vi "Tree Manager.vi"(7 "Mode":T4, 9 "Alias":string, 10 "Init Settings In":T1={"Step Values"=[], "Only Execute When Test Running"=TRUE, "Reset Sequence When Test Starts"=TRUE, "Current Sequence ID"=0, "Total Iterations"=0, "Current Step Start Timestamp"=0.0, "Number of Sequence Steps"=0, "Num of Analog Channels"=0, "Num of Digital Channels"=0, "Delay Before Starting Sequence"=0.0, "Show UI"=FALSE, "Time Remaining"=0.0, "Test Running"=FALSE, "Pause Timestamp"=0.0, "Default Analog Values"=[], "Default Digital Values"=[]}, 11 "Init Refs":T3) -> (3 "Settings Out":T1={"Step Values"=[], "Only Execute When Test Running"=TRUE, "Reset Sequence When Test Starts"=TRUE, "Current Sequence ID"=0, "Total Iterations"=0, "Current Step Start Timestamp"=0.0, "Number of Sequence Steps"=0, "Num of Analog Channels"=0, "Num of Digital Channels"=0, "Delay Before Starting Sequence"=0.0, "Show UI"=FALSE, "Time Remaining"=0.0, "Test Running"=FALSE, "Pause Timestamp"=0.0, "Default Analog Values"=[], "Default Digital Values"=[]})   [LabVIEW 2020, in "Sequencer with Output Values.lvlib" / "Sequencer with Output Values.lvclass"]
uses:
  Sequencer with Output Values.lvclass
  Tree Manager Mode.ctl
  Control Refs.ctl
  Params.ctl
  Step Settings.ctl
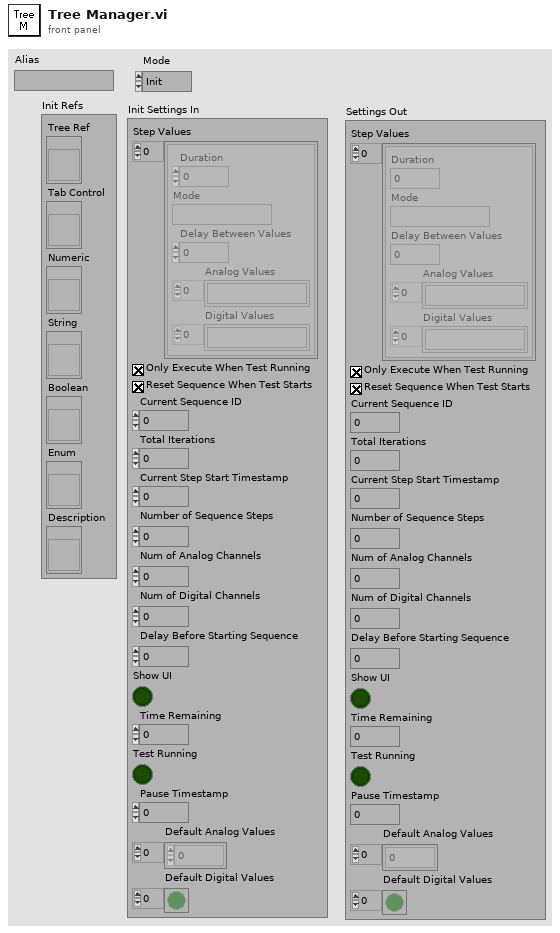
[diagram p1: front panel]
types:
  T1 = typedef "Sequencer with Output Values.lvlib/Sequencer with Output Values.lvclass/Params.ctl" = cluster{"Step Values":T2[], "Only Execute When Test Running":bool, "Reset Sequence When Test Starts":bool, "Current Sequence ID":u32, "Total Iterations":u32, "Current Step Start Timestamp":dbl, "Number of Sequence Steps":i32, "Num of Analog Channels":i32, "Num of Digital Channels":i32, "Delay Before Starting Sequence":dbl, "Show UI":bool, "Time Remaining":dbl, "Test Running":bool, "Pause Timestamp":dbl, "Default Analog Values":dbl[], "Default Digital Values":bool[]}
  T2 = typedef "Sequencer with Output Values.lvlib/Sequencer with Output Values.lvclass/Step Settings.ctl" = cluster{"Duration":dbl, "Mode":string, "Delay Between Values":dbl, "Analog Values":string[], "Digital Values":string[]}
  T3 = typedef "Sequencer with Output Values.lvlib/Sequencer with Output Values.lvclass/Control Refs.ctl" = cluster{"Tree Ref":refnum<vi>, "Tab Control":refnum<vi>, "Numeric":refnum<vi>, "String":refnum<vi>, "Boolean":refnum<vi>, "Enum":refnum<vi>, "Description":refnum<vi>}
  T4 = typedef "Sequencer with Output Values.lvlib/Sequencer with Output Values.lvclass/Tree Manager Mode.ctl" = enum16{"Init", "Tree Change", "Value Change", "Close"}
  T5 = typedef "Sequencer with Output Values.lvlib/Sequencer with Output Values.lvclass/Tree Item Settings.ctl" = cluster{"Indent Level":i32, "Data Type":T6, "Numeric Range":cluster{"Min":dbl, "Max":dbl, "Inc":dbl}, "Enum Values":string[], "Default Value":string}
  T6 = typedef "Sequencer with Output Values.lvlib/Sequencer with Output Values.lvclass/Data Type.ctl" = i16
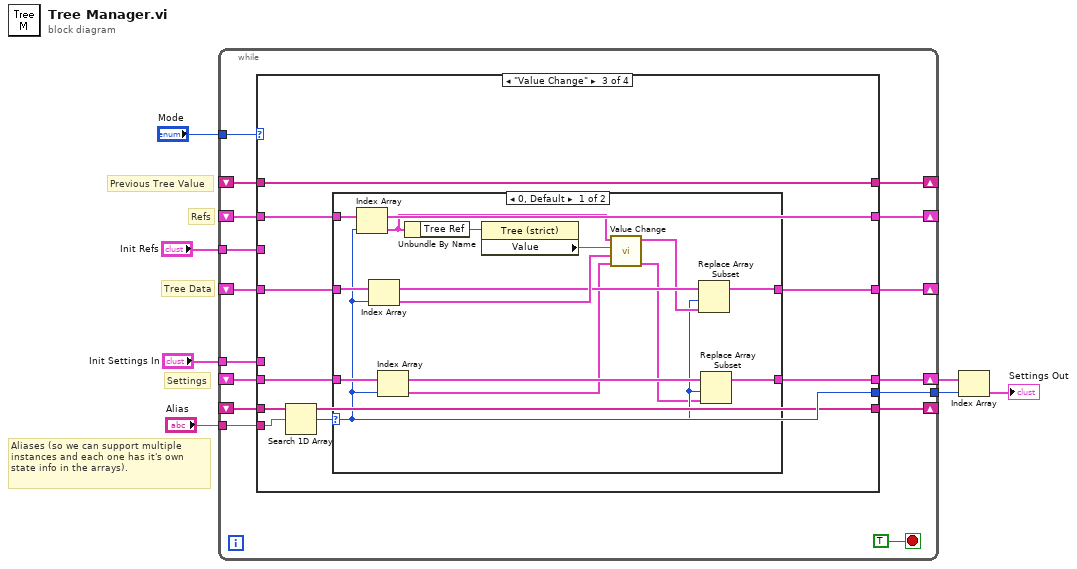
[diagram p0: block diagram]
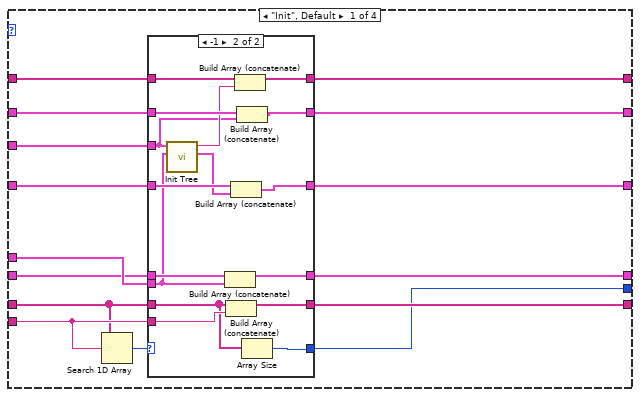
[diagram p2: hidden frame]
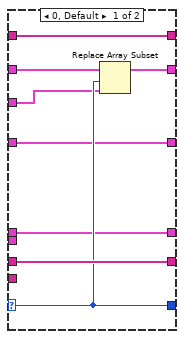
[diagram p3: hidden frame]
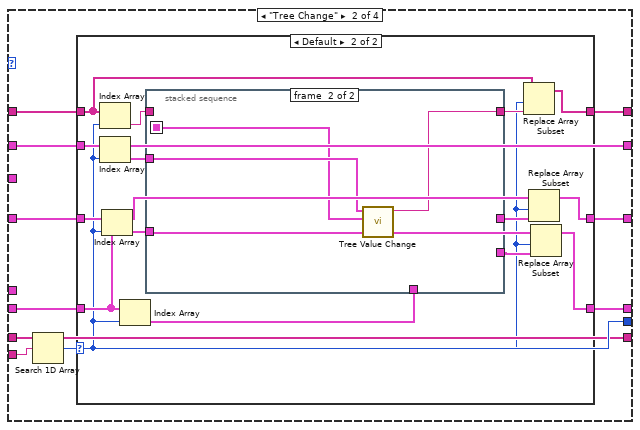
[diagram p4: hidden frame]
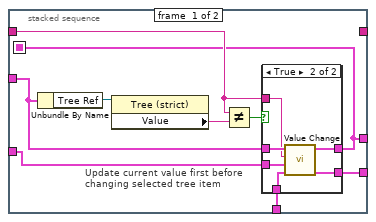
[diagram p6: hidden frame]
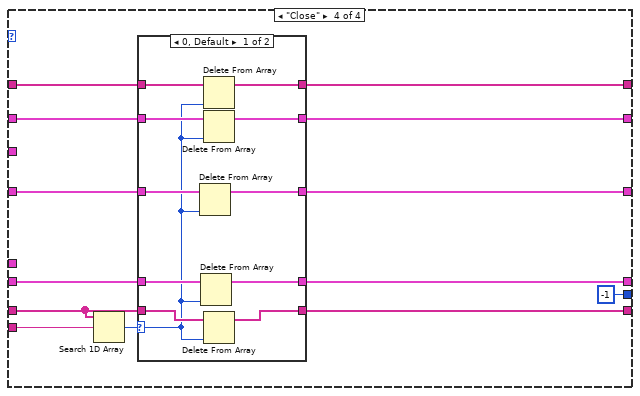
[diagram p9: hidden frame]
diagram:
  # "Aliases (so we can support multiple instances and each one has it's own state info in the arrays)."
  # "Previous Tree Value"
  # "Tree Data"
  # "Settings"
  # "Refs"
  n1 = while {
    tunnel: "Mode" -> [w23]
    tunnel: "Init Refs" -> [w22]
    tunnel: "Init Settings In" -> [w20]
    shift-right: [w19] -> _
    shift-left: _ -> [w18]
    shift-right: [w17] -> w4
    shift-left: _ -> [w16]
    shift-right: [w15] -> _
    shift-left: _ -> [w14]
    shift-right: [w13] -> _
    shift-left: _ -> [w12]
    tunnel: "Alias" -> [w11]
    shift-right: [w10] -> _
    shift-left: _ -> [w9]
    tunnel: [w8] -> w3
    stop <- TRUE stop-if-true
    n2 = case shown="\"Value Change\"" w23 {
      tunnel: w22 -> [w24 _ _ _]
      tunnel: w20 -> [w34 _ _ _]
      tunnel: [w26 w71 w118 w142] -> w19
      tunnel: w18 -> [w25 w71 w118 w143]
      tunnel: [w33 w67 w114 w138] -> w17
      tunnel: w16 -> [w32 w68 w116 w139]
      tunnel: [w30 w66 w115 w140] -> w15
      tunnel: w14 -> [w29 w72 w117 w141]
      tunnel: [w28 w70 w119 w144] -> w13
      tunnel: w12 -> [w27 w69 w119 w145]
      tunnel: w11 -> [w37 w65 w113 w147]
      tunnel: [w38 w63 w111 w136] -> w10
      tunnel: w9 -> [w35 w63 w111 w137]
      tunnel: [w31 w64 w112 -1 ("index of element")] -> w8
      frame "Init", Default {
        n3 = Search 1D Array(1D array=w35, element=w37) -> (index of element=w36:i32)  [unwired: 1 in]
        n4 = case shown="-1" w36 {
          selector: w36 -> [w43 _]
          tunnel: [w46 w62] -> w38
          tunnel: w37 -> [_ w61]
          tunnel: w35 -> [w46 w58]
          tunnel: w34 -> [_ w50]
          tunnel: [w39 w60] -> w33
          tunnel: w32 -> [w39 w59]
          tunnel: [w43 w57] -> w31
          tunnel: [w40 w56] -> w30
          tunnel: w29 -> [w40 w55]
          tunnel: [w42 w54] -> w28
          tunnel: w27 -> [w42 w53]
          tunnel: [w44 w52] -> w26
          tunnel: w25 -> [w45 w51]
          tunnel: w24 -> [w41 w47]
          frame 0, Default {
            n5 = Replace Array Subset(array=w45, new element=w41, index=w43) -> (w44:T3[])
          }
          frame -1 {
            n6 = call "Init Tree.vi"("Settings In"=w50, "Init Refs"=w47) -> ("Tree Data"=w48:cluster{string[], T5[]}, "Selected Tag"=w49:string)  [unwired: 8 in]
            n7 = Build Array (concatenate)(w59, w50) -> (w60:T1[])
            n8 = Build Array (concatenate)(w58, w61) -> (w62:string[])
            n9 = Build Array (concatenate)(w55, w48) -> (w56:cluster{string[], T5[]}[])
            n10 = Build Array (concatenate)(w53, w49) -> (w54:string[])
            n11 = Build Array (concatenate)(w51, w47) -> (w52:T3[])
            n12 = Array Size(array=w58) -> (size(s)=w57:i32)
          }
        }
      }
      frame "Tree Change" {
        n13 = Search 1D Array(1D array=w63, element=w65) -> (index of element=w64:i32)  [unwired: 1 in]
        n14 = case shown="Default" w64 {
          selector: w64 -> [_ w77]
          tunnel: w72 -> [w74 w82]
          tunnel: w71 -> [_ w90]
          tunnel: [w75 w83] -> w70
          tunnel: w69 -> [w75 w85]
          tunnel: w68 -> [w73 w79]
          tunnel: [w73 w76] -> w67
          tunnel: [w74 w80] -> w66
          frame -1 {
          }
          frame Default {
            n15 = Index Array(array=w85, index=w77) -> (element=w88:string)
            n16 = Index Array(array=w90, index=w77) -> (element=w89:T3)
            n17 = Index Array(array=w82, index=w77) -> (element=w87:cluster{string[], T5[]})
            n18 = Index Array(array=w79, index=w77) -> (element=w86:T1)
            n19 = stacked-sequence {
              seq-local: [w91 _] -> [_ w108]
              tunnel: w87 -> [w94 _]
              tunnel: w89 -> [w98 w110]
              tunnel: [_ w109] -> w84
              tunnel: w88 -> [w95 _]
              tunnel: w86 -> [w93 _]
              tunnel: [w92 _] -> w78
              tunnel: [w91 _] -> w81
              frame #0 {
                # "Update current value first before changing selected tree item"
                n20 = Unbundle By Name(w98) -> ("Tree Ref"=w99:refnum<vi>)
                n21 = property class="Tree (strict)"(reference=w99) -> ("Value"=w97:string)  [unwired: 1 in, 2 out]
                n22 = Not Equal?(x=w95, y=w97) -> (x != y?=w96:bool)
                n23 = case shown="True" w96 {
                  tunnel: w98 -> [_ w107]
                  tunnel: w95 -> [_ w106]
                  tunnel: w94 -> [w101 w105]
                  tunnel: w93 -> [w100 w104]
                  tunnel: [w101 w103] -> w91
                  tunnel: [w100 w102] -> w92
                  frame False {
                  }
                  frame True {
                    n24 = call "Value Change.vi"("Settings In"=w104, "Tree Data"=w105, "Tree Tag"=w106, "Init Refs"=w107) -> ("Settings Out"=w102:T1, "Tree Data out"=w103:cluster{"Tag":string[], "Settings":T5[]})  [unwired: 6 in]
                  }
                }
              }
              frame #1 {
                n25 = call "Tree Value Change.vi"("Tree Data"=w108, "Init Refs"=w110) -> ("Value"=w109:string)  [unwired: 9 in]
              }
            }
            n26 = Replace Array Subset(array=w85, new element=w84, index=w77) -> (w83:string[])
            n27 = Replace Array Subset(array=w82, new element=w81, index=w77) -> (w80:cluster{string[], T5[]}[])
            n28 = Replace Array Subset(array=w79, new element=w78, index=w77) -> (w76:T1[])
          }
        }
      }
      frame "Value Change" {
        n29 = Search 1D Array(1D array=w111, element=w113) -> (index of element=w112:i32)  [unwired: 1 in]
        n30 = case shown="0, Default" w112 {
          selector: w112 -> [w122 _]
          tunnel: w118 -> [w130 _]
          tunnel: w117 -> [w128 w134]
          tunnel: w116 -> [w125 w133]
          tunnel: [w126 w134] -> w115
          tunnel: [w124 w133] -> w114
          frame 0, Default {
            n31 = Index Array(array=w130, index=w122) -> (element=w123:T3)
            n32 = Index Array(array=w128, index=w122) -> (element=w129:cluster{string[], T5[]})
            n33 = Index Array(array=w125, index=w122) -> (element=w121:T1)
            n34 = Unbundle By Name(w123) -> ("Tree Ref"=w132:refnum<vi>)
            n35 = property class="Tree (strict)"(reference=w132) -> ("Value"=w131:string)  [unwired: 1 in, 2 out]
            n36 = call "Value Change.vi"("Settings In"=w121, "Tree Data"=w129, "Tree Tag"=w131, "Init Refs"=w123) -> ("Settings Out"=w120:T1, "Tree Data out"=w127:cluster{"Tag":string[], "Settings":T5[]})  [unwired: 6 in]
            n37 = Replace Array Subset(array=w128, new element=w127, index=w122) -> (w126:cluster{string[], T5[]}[])
            n38 = Replace Array Subset(array=w125, new element=w120, index=w122) -> (w124:T1[])
          }
          frame -1 {
          }
        }
      }
      frame "Close" {
        n39 = Search 1D Array(1D array=w137, element=w147) -> (index of element=w146:i32)  [unwired: 1 in]
        n40 = case shown="0, Default" w146 {
          selector: w146 -> [w148 _]
          tunnel: w145 -> [w158 w163]
          tunnel: [w157 w163] -> w144
          tunnel: w143 -> [w156 w162]
          tunnel: [w155 w162] -> w142
          tunnel: w141 -> [w154 w161]
          tunnel: [w153 w161] -> w140
          tunnel: w139 -> [w152 w160]
          tunnel: [w151 w160] -> w138
          tunnel: w137 -> [w150 w159]
          tunnel: [w149 w159] -> w136
          frame 0, Default {
            n41 = Delete From Array(array=w154, index=w148) -> (array with subset deleted=w153:cluster{string[], T5[]}[])  [unwired: 1 in, 1 out]
            n42 = Delete From Array(array=w152, index=w148) -> (array with subset deleted=w151:T1[])  [unwired: 1 in, 1 out]
            n43 = Delete From Array(array=w158, index=w148) -> (array with subset deleted=w157:string[])  [unwired: 1 in, 1 out]
            n44 = Delete From Array(array=w156, index=w148) -> (array with subset deleted=w155:T3[])  [unwired: 1 in, 1 out]
            n45 = Delete From Array(array=w150, index=w148) -> (array with subset deleted=w149:string[])  [unwired: 1 in, 1 out]
          }
          frame -1 {
          }
        }
      }
    }
  }
  n46 = Index Array(array=w4, index=w3) -> (element=→"Settings Out":T1)
